vi "Measurement UI.vi"() -> ()   [LabVIEW 2021, in "ImageStreamRendering.lvlib"]
uses:
  ImageStreamRendering.lvlib
  <vilib>/vision/Image Controls.llb/IMAQ Image.ctl
  nivision.dll
  nivissvc.dll
panel:
  out "Image Res megapixel":dbl
  in  "External Display":bool
  out "Average Time to receive image frame":dbl
  out "Time taken to receive image frame":dbl
  out "Image Acq time":string
  out "Display Frames per Second (approx)":u32
  out "Last Buffer Number":u32
  out "Time to convert back to Image (s)":dbl
  in  "Border Size":i32=3
  in  "Image Name":string="copy"
  in  "Image Type":u32(ring)=4 items=["Grayscale (U8)", "Grayscale (I16)", "Grayscale (SGL)", "Complex (CSG)", "RGB (U32)", "HSL (U32)", "RGB (U64)", "Grayscale (U16)"]
  out "Image Resolution":i32[](array[numeric])
  in  "Camera name":string
  out "Image Pixels (U32)":u32[](array[numeric])
  in  "Image Pixels (U64) 2":T1[][](array[typedef])
  in  "Image Converison Type":string(combo)="ImagePixelArray"
  out "Image Data Received":string
  out "value":u32[][](array[numeric])
  out "Image":T2(plugin-control)
  out "error out":errorcluster
  out "Image Data":string
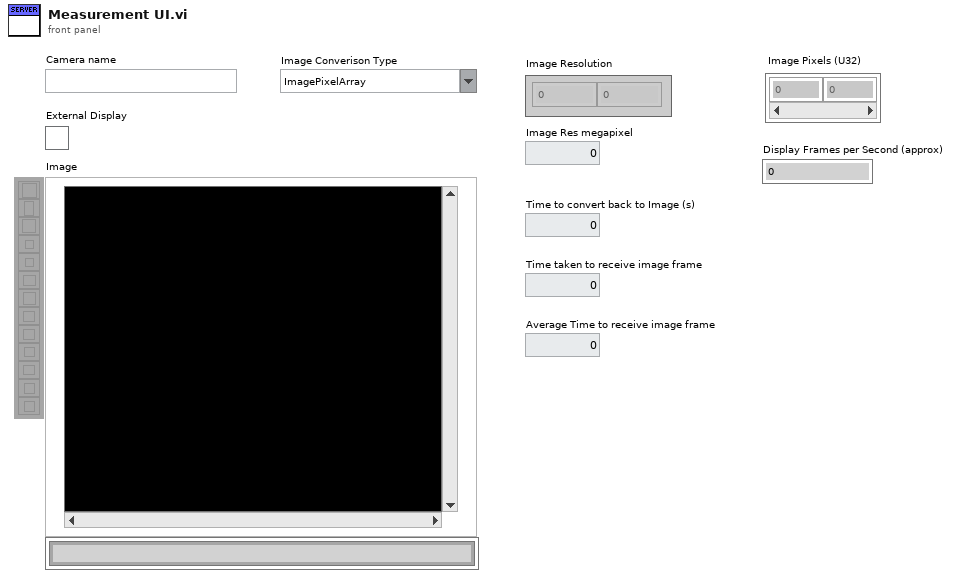
[diagram p1: front panel]
types:
  T1 = typedef "Color (U64)" = cluster{"Plane 3 (Blue)":u16, "Plane 2 (Green)":u16, "Plane 1 (Red)":u16, "Plane 4 (alpha)":u16}
  T2 = typedef "IMAQ Image.ctl" = refnum<image>
  T3 = cluster{"New Image":T2, "Run start time":timestamp, "Last Buffer Number":u32, "Time to receive image":dbl[]}
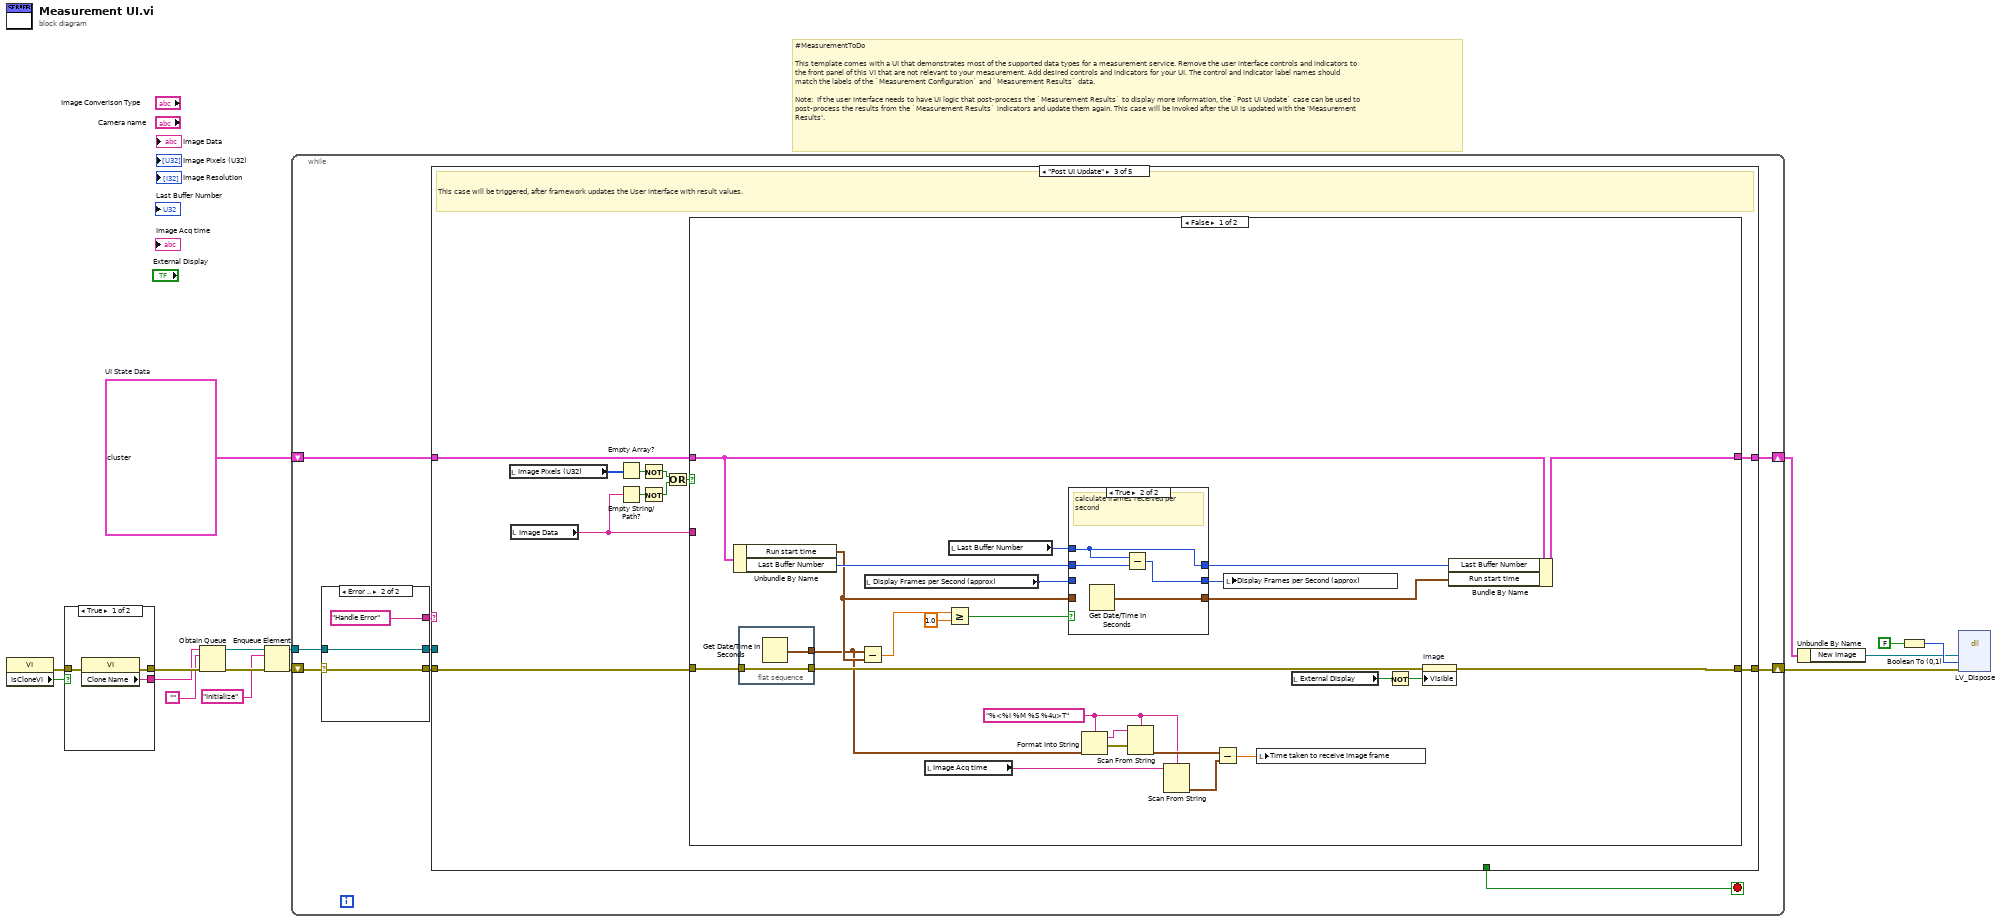
[diagram p0: block diagram]
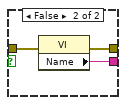
[diagram p2: hidden frame]
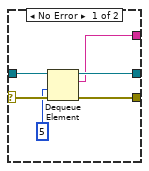
[diagram p3: hidden frame]
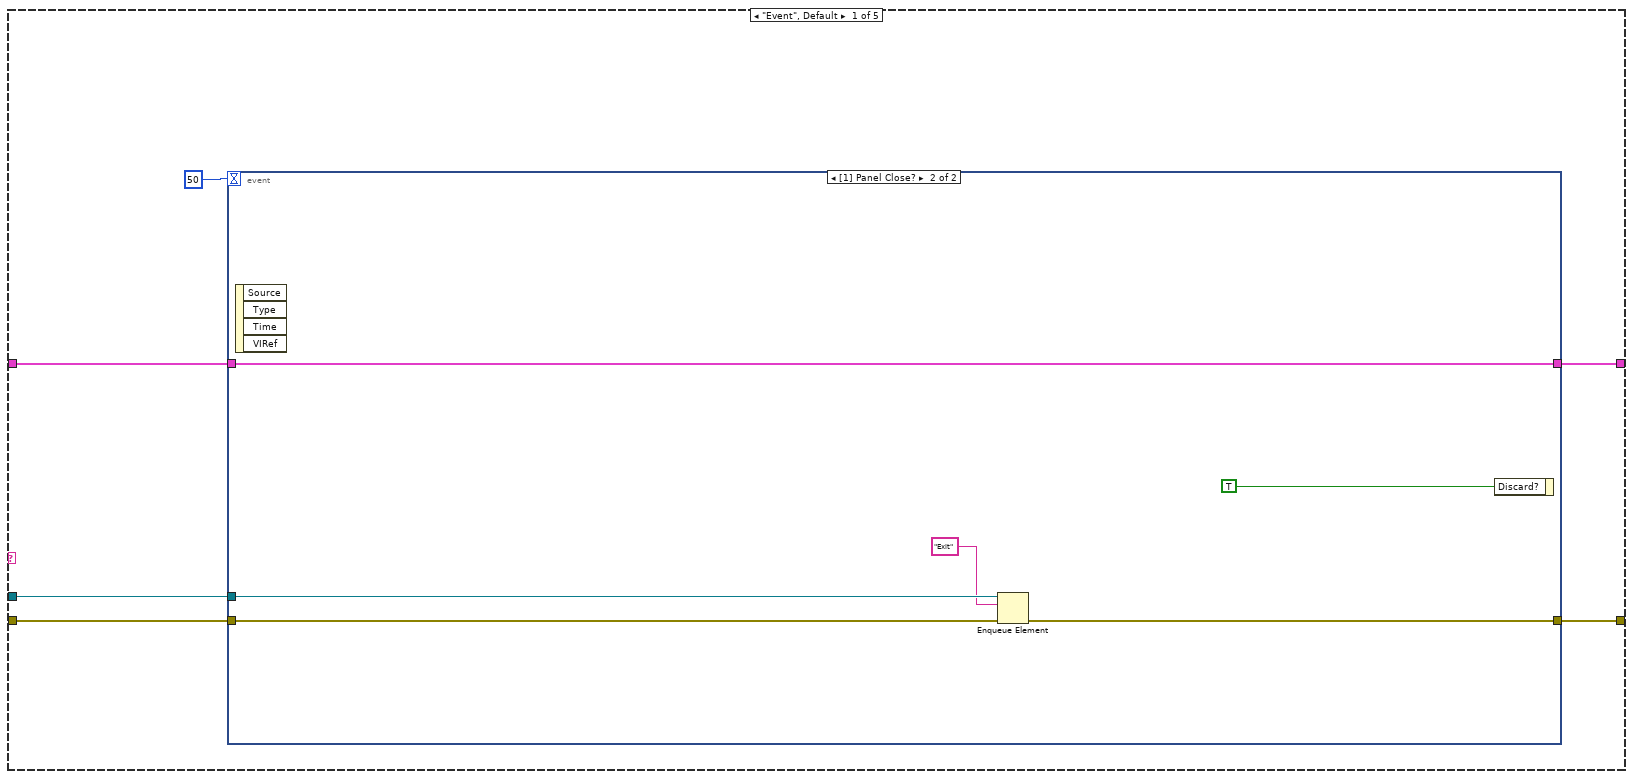
[diagram p4: hidden frame]
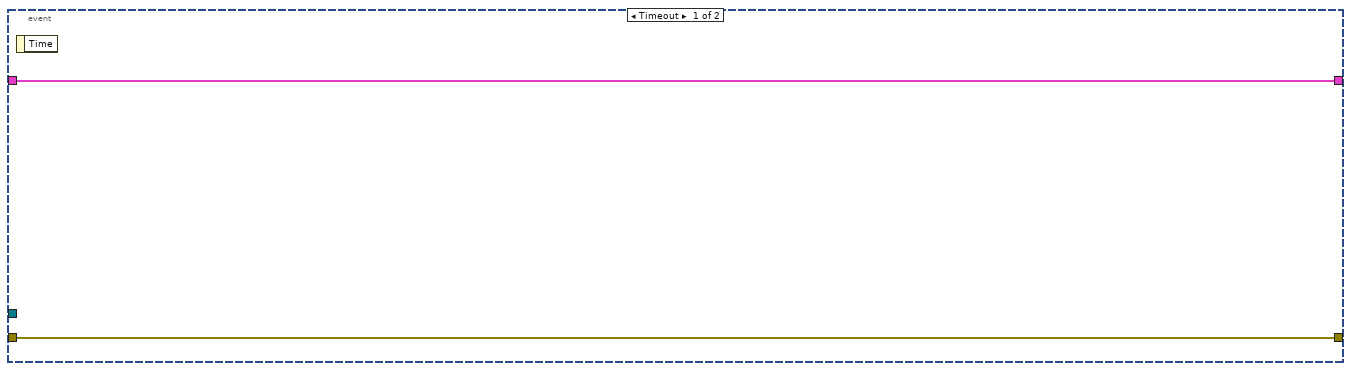
[diagram p5: hidden frame]
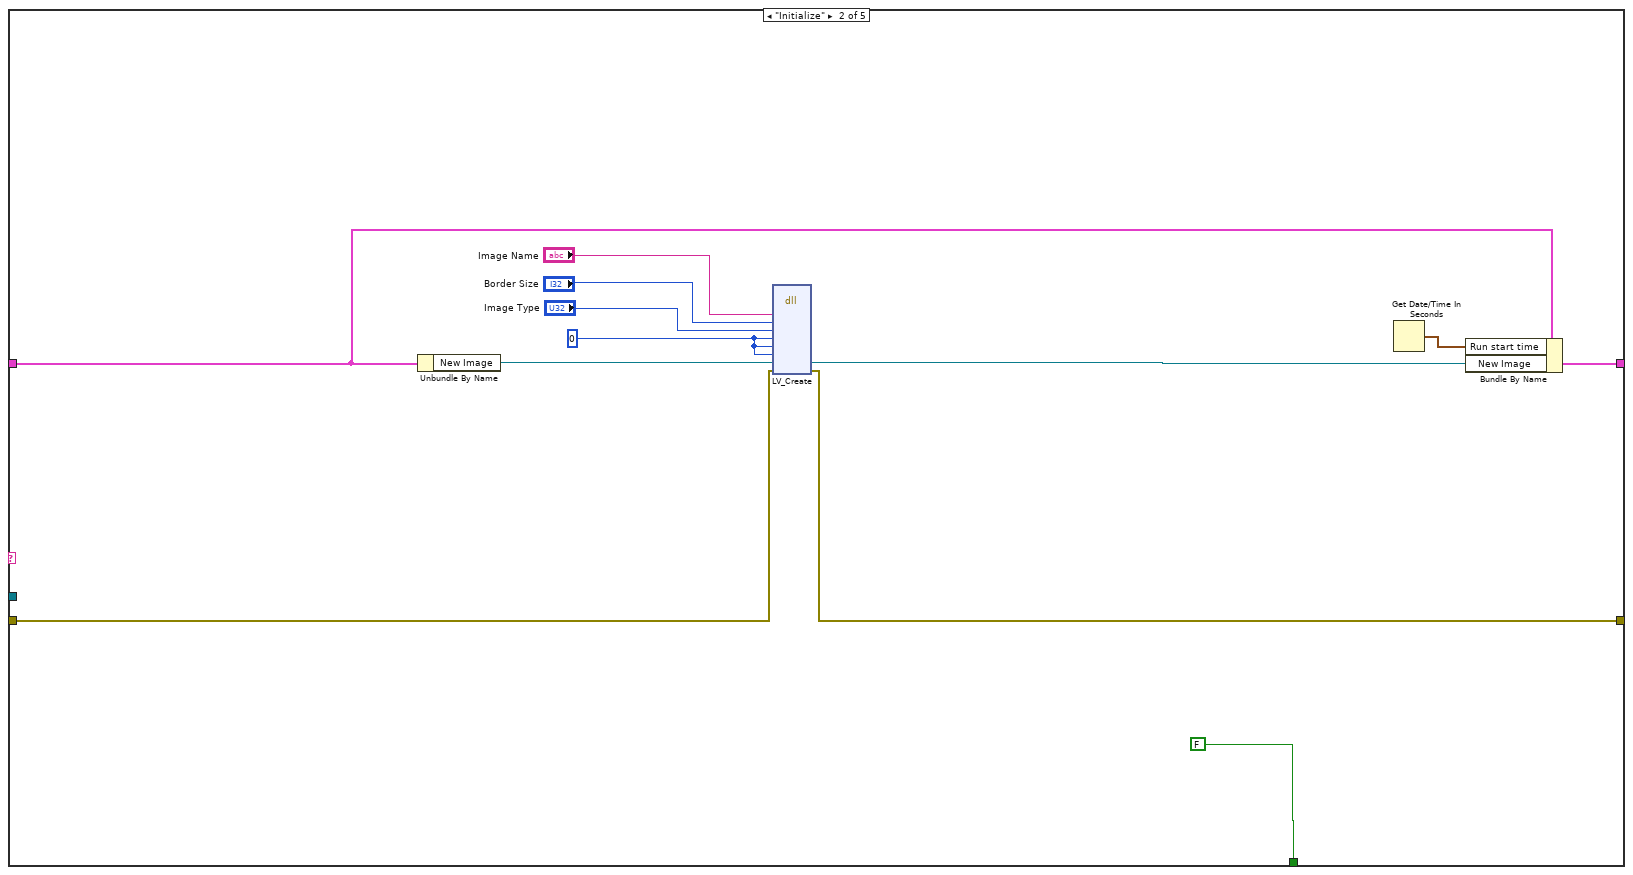
[diagram p6: hidden frame]
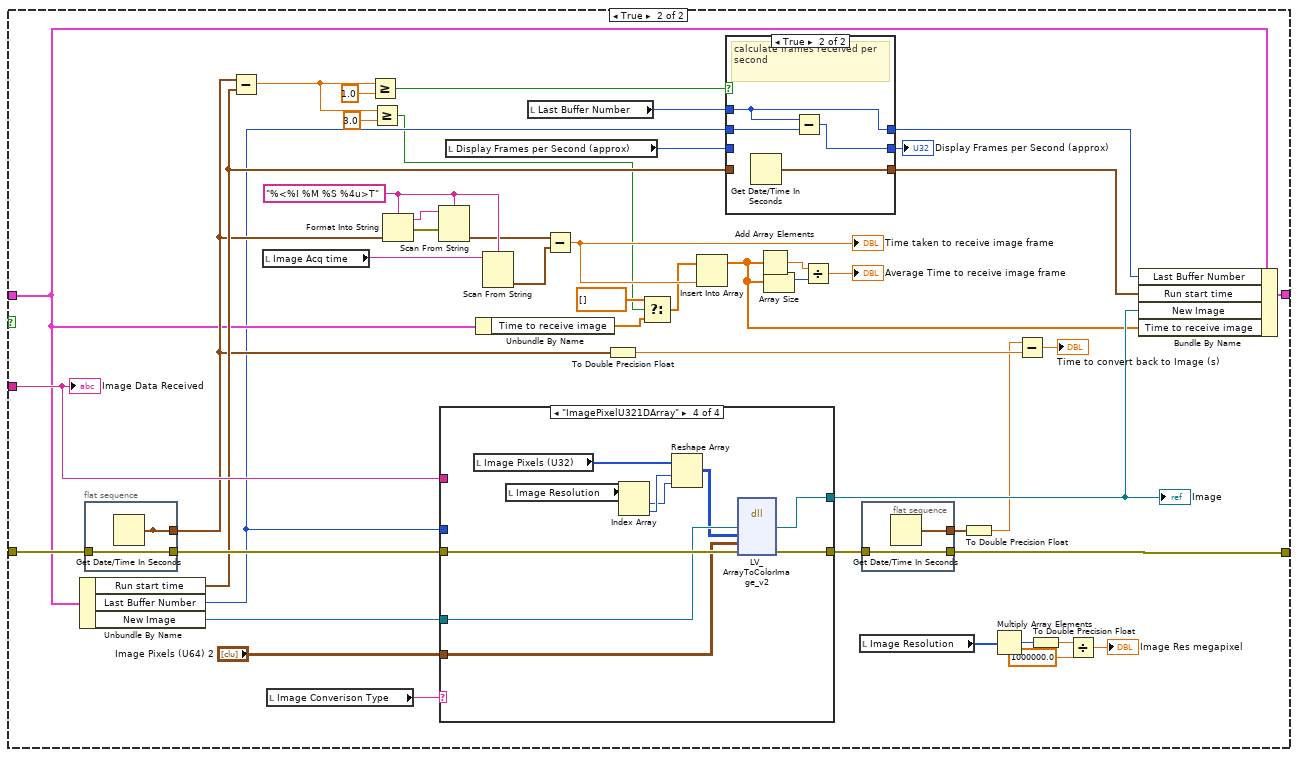
[diagram p8: hidden frame]
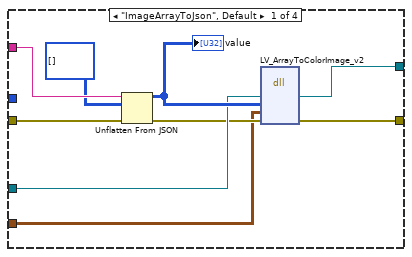
[diagram p10: hidden frame]
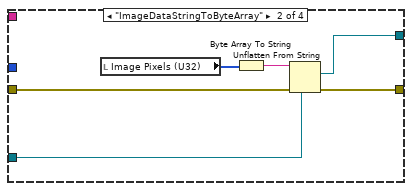
[diagram p11: hidden frame]
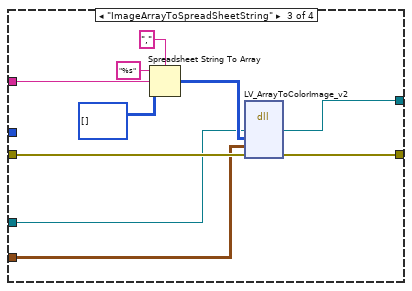
[diagram p12: hidden frame]
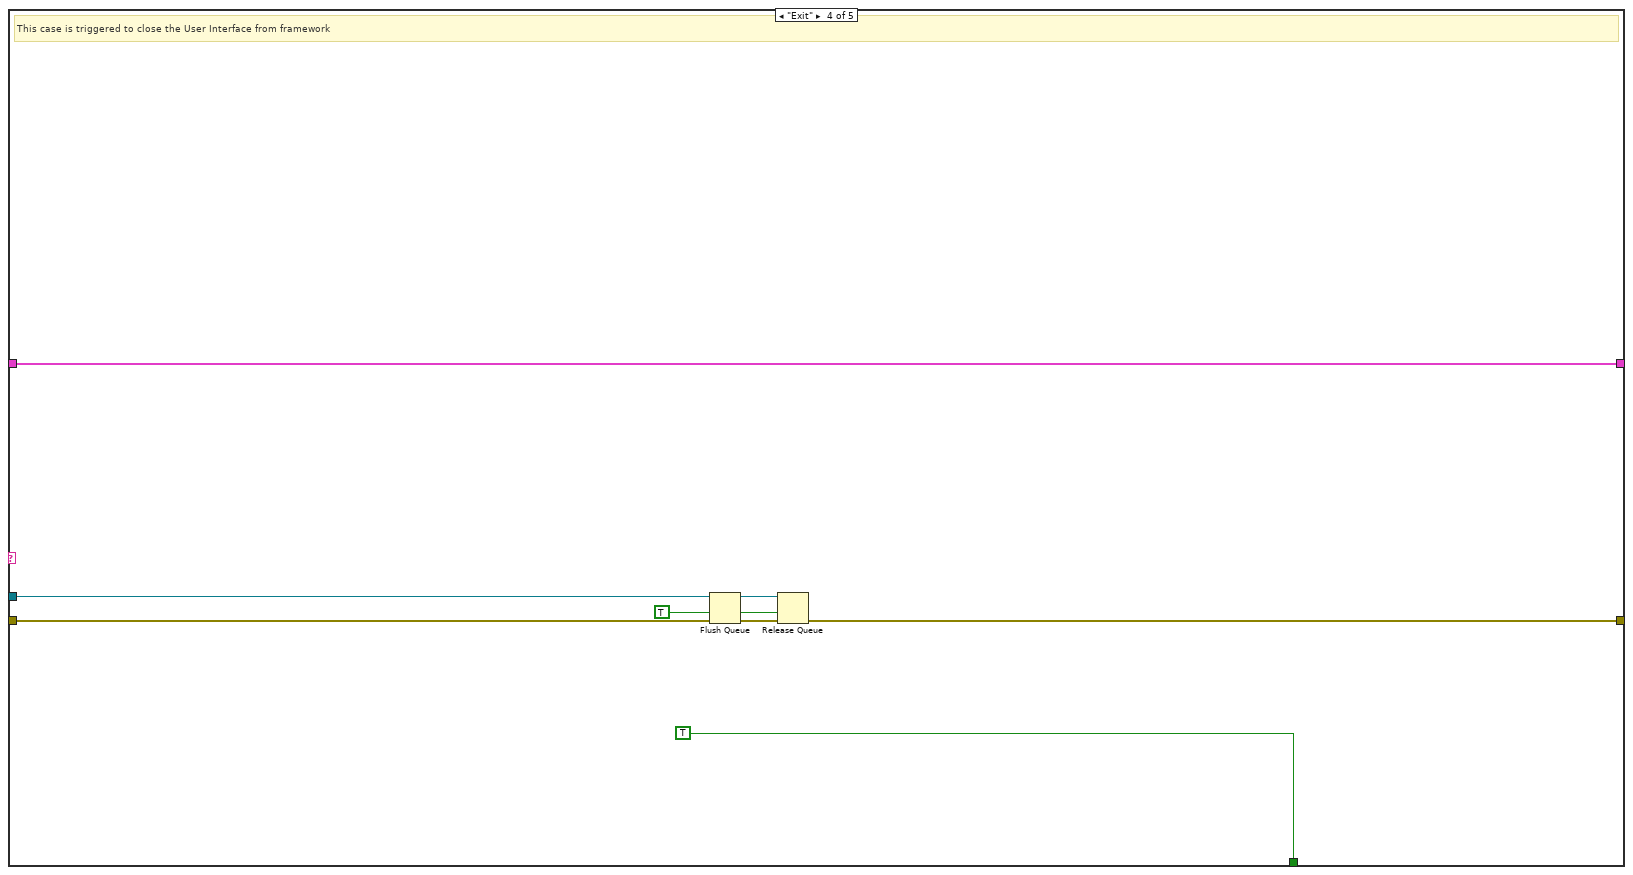
[diagram p13: hidden frame]
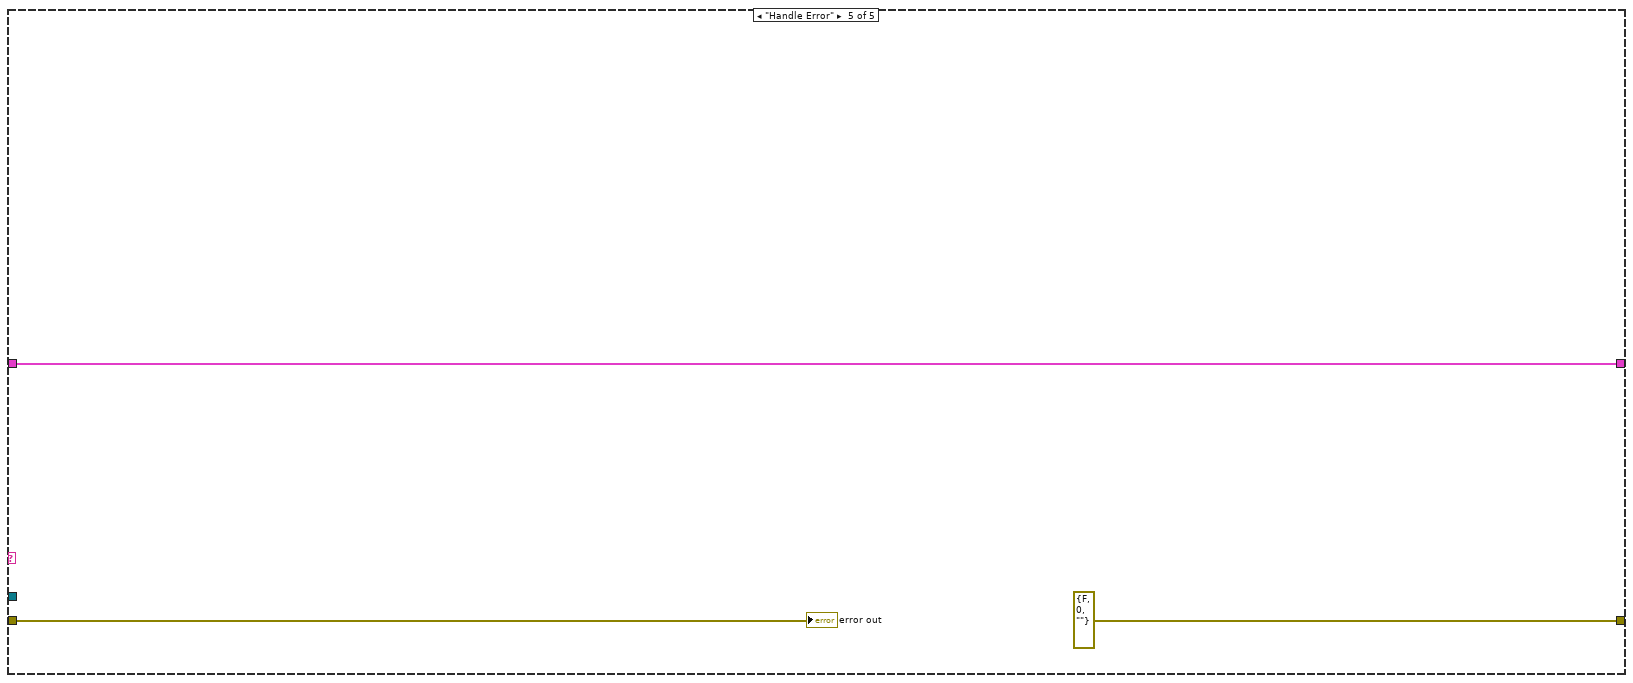
[diagram p14: hidden frame]
diagram:
  w2 = T3 {"New Image"=refnum, "Run start time"=timestamp(0 s since 1904-01-01), "Last Buffer Number"=0, "Time to receive image"=[]}  # UI State Data
  # "#MeasurementToDo  \n\nThis template comes with a UI that demonstrates most of the supported data types for a measurement service. Remove the user interface controls and indicators to the front panel of this VI that are not relevant to your measurement. Add desired controls and indicators for your UI. The control and indicator label names should match the labels of the `Measurement Configuration` and `Measurement Results` data.\n\nNote:  If the user interface needs to have UI logic that post-process the `Measurement Results` to display more information, the `Post UI Update` case can be used to post-process the results from the `Measurement Results` indicators and update them again. This case will be invoked after the UI is updated with the 'Measurement Results'."
  n1 = property class="VI"() -> (error out=w7:errorcluster, "IsCloneVI"=w8:bool)  [unwired: 2 in, 1 out]
  n2 = case shown="True" w8 {
    tunnel: [w19 w22] -> w16
    tunnel: [w18 w21] -> w15
    tunnel: w7 -> [w17 w20]
    frame True {
      n3 = property class="VI"(error in=w17) -> (error out=w19:errorcluster, "Clone Name"=w18:string)  [unwired: 1 in, 1 out]
    }
    frame False {
      n4 = property class="VI"(error in=w20) -> (error out=w22:errorcluster, "Name"=w21:string)  [unwired: 1 in, 1 out]
    }
  }
  n5 = Obtain Queue(name (unnamed)=w15, element data type="", error in (no error)=w16) -> (queue out=w12:refnum<queue>, error out=w14:errorcluster)  [unwired: 2 in, 1 out]
  n6 = Enqueue Element(queue=w12, element="Initialize", error in (no error)=w14) -> (queue out=w11:refnum<queue>, error out=w13:errorcluster)  [unwired: 1 in, 1 out]
  n7 = while {
    shift-right: [w27] -> w5
    shift-left: w13 -> [w31]
    tunnel: w11 -> [w30]
    shift-right: [w24] -> w3
    shift-left: w2 -> [w23]
    stop <- w26 stop-if-true
    n8 = case shown="Error .." w31 {
      selector: w31 -> [w37 w40]
      tunnel: [w36 w40] -> w25
      tunnel: w30 -> [w35 w39]
      tunnel: [w34 w39] -> w29
      tunnel: [w33 "Handle Error"] -> w28
      frame No Error {
        n9 = Dequeue Element(queue=w35, timeout in ms (-1)=5, error in (no error)=w37) -> (queue out=w34:refnum<queue>, element=w33:string, error out=w36:errorcluster)  [unwired: 1 out]
      }
      frame Error {
      }
    }
    n10 = case shown="\"Post UI Update\"" w28 {
      tunnel: w25 -> [w45 w61 w67 w212 w215]
      tunnel: w29 -> [w43 _ _ w210 _]
      tunnel: [w46 w55 w77 w207 errorcluster {"status"=FALSE, "code"=0, "source"=""} ("error out")] -> w27
      tunnel: [_ FALSE _ TRUE _] -> w26
      tunnel: [w41 w58 w69 w205 w214] -> w24
      tunnel: w23 -> [w42 w57 w68 w205 w214]
      frame "Event", Default {
        n11 = event shown="[1] Panel Close?" {
          selector: _ -> [_ _]
          dyn-events: _ -> [_ _]
          timeout: 50 -> [_ _]
          tunnel: [w48 w52] -> w46
          tunnel: w45 -> [w48 w53]
          tunnel: w43 -> [_ w51]
          tunnel: w42 -> [w47 w49]
          tunnel: [w47 w49] -> w41
          event Timeout {
            n12 = event-data() -> ()  [unwired: 1 in, 1 out]
          }
          event Panel Close? {
            n13 = event-data() -> ()  [unwired: 1 in, 4 out]
            n14 = Enqueue Element(queue=w51, element="Exit", error in (no error)=w53) -> (error out=w52:errorcluster)  [unwired: 1 in, 2 out]
            n15 = event-data("Discard?"=TRUE) -> ()  [unwired: 1 in, 1 out]
          }
        }
      }
      frame "Initialize" {
        w62 = 0
        n16 = Unbundle By Name(w57) -> ("New Image"=w59:T2)
        n17 = dll-call lib="nivissvc.*" fn="LV_Create" label="Imaq Create"("name"="Image Name", "border"="Border Size", "imageType"="Image Type", "width"=w62, "height"=w62, "lock space"=w62, "image"=w59, "error out 2"=w61) -> ("image"=w60:T2, "error out 2"=w55:errorcluster)  [unwired: 9 in, 3 out]
        n18 = Get Date/Time In Seconds() -> (seconds since 1Jan1904=w56:timestamp)
        n19 = Bundle By Name(cluster=w57, "Run start time"=w56, "New Image"=w60) -> (w58:T3)
      }
      frame "Post UI Update" {
        # "This case will be triggered, after framework updates the User interface with result values."
        n20 = local read "Image Pixels (U32)"() -> (w75:u32[])
        n21 = local read "Image Data"() -> (w73:string)
        n22 = Empty Array?(array=w75) -> (empty?=w76:bool)
        n23 = Empty String/Path?(string/path=w73) -> (empty?=w72:bool)
        n24 = Not(x=w76) -> (.not. x?=w74:bool)
        n25 = Not(x=w72) -> (.not. x?=w71:bool)
        n26 = Or(x=w74, y=w71) -> (x .or. y?=w70:bool)
        n27 = case shown="False" w70 {
          tunnel: [w100 w153] -> w77
          tunnel: w67 -> [w98 w157]
          tunnel: w73 -> [_ w155]
          tunnel: [w88 w149] -> w69
          tunnel: w68 -> [w99 w128]
          frame False {
            w81 = "%<%I %M %S %4u>T" ("format string")
            n28 = Unbundle By Name(w99) -> ("Run start time"=w92:timestamp, "Last Buffer Number"=w96:u32)
            n29 = flat-sequence {
              tunnel: w98 -> [w104]
              tunnel: [w104] -> w97
              tunnel: [w103] -> w79
              frame #0 {
                n30 = Get Date/Time In Seconds() -> (seconds since 1Jan1904=w103:timestamp)
              }
            }
            n31 = Subtract(x=w79, y=w92) -> (x-y=w94:dbl)
            n32 = local read "Display Frames per Second (approx)"() -> (w90:u32)
            n33 = local read "Image Acq time"() -> (w80:string)
            n34 = Greater Or Equal?(x=w94, y=1.0) -> (x >= y?=w93:bool)
            n35 = local read "Last Buffer Number"() -> (w91:u32)
            n36 = case shown="True" w93 {
              tunnel: w96 -> [w105 w111]
              tunnel: [w107 w110] -> w86
              tunnel: w92 -> [w107 _]
              tunnel: [w106 w109] -> w89
              tunnel: w90 -> [w106 _]
              tunnel: w91 -> [_ w108]
              tunnel: [w105 w108] -> w87
              frame False {
              }
              frame True {
                # "calculate frames received per second"
                n37 = Get Date/Time In Seconds() -> (seconds since 1Jan1904=w110:timestamp)
                n38 = Subtract(x=w108, y=w111) -> (x-y=w109:u32)
              }
            }
            n39 = Format Into String(format string=w81, w79) -> (resulting string=w83:string, error out=w84:errorcluster)  [unwired: 2 in]
            n40 = Scan From String(format string=w81, input string=w83, error in=w84) -> (output 1=w82:timestamp)  [unwired: 2 in, 3 out]
            n41 = Scan From String(format string=w81, input string=w80) -> (output 1=w85:timestamp)  [unwired: 3 in, 3 out]
            n42 = Subtract(x=w82, y=w85) -> (x-y=w78:dbl)
            n43 = local write "Display Frames per Second (approx)"(w89) -> ()
            n44 = local write "Time taken to receive image frame"(w78) -> ()
            n45 = local read "External Display"() -> (w101:bool)
            n46 = Not(x=w101) -> (.not. x?=w102:bool)
            n47 = property on="Image" class="ImageControl"(error in=w97, "Visible"=w102) -> (error out=w100:errorcluster)  [unwired: 1 in, 1 out]
            n48 = Bundle By Name(cluster=w99, "Last Buffer Number"=w87, "Run start time"=w86) -> (w88:T3)
          }
          frame True {
            w138 = "%<%I %M %S %4u>T" ("format string")
            n49 = Unbundle By Name(w128) -> ("Run start time"=w144:timestamp, "Last Buffer Number"=w125:u32, "New Image"=w132:T2)
            n50 = flat-sequence {
              tunnel: w157 -> [w202]
              tunnel: [w202] -> w152
              tunnel: [w201] -> _
              tunnel: [w201] -> w133
              frame #0 {
                n51 = Get Date/Time In Seconds() -> (seconds since 1Jan1904=w201:timestamp)
              }
            }
            n52 = Subtract(x=w133, y=w144) -> (x-y=w117:dbl)
            n53 = local read "Image Acq time"() -> (w142:string)
            n54 = local read "Image Converison Type"() -> (w156:string)
            n55 = Greater Or Equal?(x=w117, y=1.0) -> (x >= y?=w147:bool)
            n56 = Greater Or Equal?(x=w117, y=3.0) -> (x >= y?=w113:bool)
            n57 = Format Into String(format string=w138, w133) -> (resulting string=w139:string, error out=w140:errorcluster)  [unwired: 2 in]
            n58 = Scan From String(format string=w138, input string=w139, error in=w140) -> (output 1=w137:timestamp)  [unwired: 2 in, 3 out]
            n59 = case shown="\"ImagePixelU321DArray\"" w156 {
              tunnel: w155 -> [w174 _ w190 _]
              tunnel: w132 -> [w171 w178 w183 w198]
              tunnel: [w170 w177 w182 w197] -> w131
              tunnel: [w169 w179 w186 w199] -> w158
              tunnel: w152 -> [w168 w180 w187 w200]
              tunnel: "Image Pixels (U64) 2" -> [w166 _ w181 w196]
              tunnel: w125 -> [_ _ _ _]
              frame "ImageArrayToJson", Default {
                n60 = Unflatten From JSON(JSON string=w174, type and defaults=u32[][] [] ("Image Pixels (U32)"), error in (no error)=w168) -> (value=w172:u32[][], error out=w167:errorcluster)  [unwired: 4 in]
                "value" <- w172
                n61 = dll-call lib="nivision.*" fn="LV_ArrayToColorImage_v2"("image"=w171, "array32"=w172, "array64"=w166, "error"=w167) -> ("image"=w170:T2, "error"=w169:errorcluster)  [unwired: 5 in, 3 out]
              }
              frame "ImageDataStringToByteArray" {
                n62 = local read "Image Pixels (U32)"() -> (w176:u32[])
                n63 = Byte Array To String(unsigned byte array=w176) -> (string=w175:string)
                n64 = Unflatten From String(type=w178, binary string=w175, error in (no error)=w180) -> (value=w177:T2, error out=w179:errorcluster)  [unwired: 2 in, 1 out]
              }
              frame "ImageArrayToSpreadSheetString" {
                n65 = Spreadsheet String To Array(delimiter (Tab)=",", format string="%s", spreadsheet string=w190, array type (2D Dbl)=u32[][] [] ("Image Pixels (U32)")) -> (array=w185:u32[][])
                n66 = dll-call lib="nivision.*" fn="LV_ArrayToColorImage_v2"("image"=w183, "array32"=w185, "array64"=w181, "error"=w187) -> ("image"=w182:T2, "error"=w186:errorcluster)  [unwired: 5 in, 3 out]
              }
              frame "ImagePixelU321DArray" {
                n67 = local read "Image Pixels (U32)"() -> (w195:u32[])
                n68 = local read "Image Resolution"() -> (w194:i32[])
                n69 = Index Array(array=w194) -> (element #1=w192:i32, element #2=w193:i32)  [unwired: 2 in]
                n70 = Reshape Array(w195, w193, w192) -> (w191:u32[][])
                n71 = dll-call lib="nivision.*" fn="LV_ArrayToColorImage_v2"("image"=w198, "array32"=w191, "array64"=w196, "error"=w200) -> ("image"=w197:T2, "error"=w199:errorcluster)  [unwired: 5 in, 3 out]
              }
            }
            "Image" <- w131
            n72 = local read "Display Frames per Second (approx)"() -> (w145:u32)
            n73 = Unbundle By Name(w128) -> ("Time to receive image"=w115:dbl[])
            n74 = Scan From String(format string=w138, input string=w142) -> (output 1=w141:timestamp)  [unwired: 3 in, 3 out]
            n75 = local read "Last Buffer Number"() -> (w146:u32)
            n76 = Subtract(x=w137, y=w141) -> (x-y=w127:dbl)
            "Time taken to receive image frame" <- w127
            n77 = To Double Precision Float(number=w133) -> (double precision float=w119:dbl)
            n78 = Select(t=dbl[] [], s=w113, f=w115) -> (s? t:f=w112:dbl[])
            n79 = Insert Into Array(array=w112, new element=w127) -> (w126:dbl[])  [unwired: 1 in]
            n80 = case shown="True" w147 {
              tunnel: w125 -> [w159 w165]
              tunnel: [w161 w164] -> w129
              tunnel: w144 -> [w161 _]
              tunnel: [w160 w163] -> w143
              tunnel: w145 -> [w160 _]
              tunnel: w146 -> [_ w162]
              tunnel: [w159 w162] -> w130
              frame False {
              }
              frame True {
                # "calculate frames received per second"
                n81 = Get Date/Time In Seconds() -> (seconds since 1Jan1904=w164:timestamp)
                n82 = Subtract(x=w162, y=w165) -> (x-y=w163:u32)
              }
            }
            "Display Frames per Second (approx)" <- w143
            n83 = Add Array Elements(numeric array=w126) -> (sum=w136:dbl)
            n84 = Array Size(array=w126) -> (size(s)=w135:i32)
            n85 = Divide(x=w136, y=w135) -> (x/y=→"Average Time to receive image frame":dbl)
            n86 = local read "Image Resolution"() -> (w124:i32[])
            n87 = flat-sequence {
              tunnel: w158 -> [w204]
              tunnel: [w204] -> w153
              tunnel: [w203] -> w151
              frame #0 {
                n88 = Get Date/Time In Seconds() -> (seconds since 1Jan1904=w203:timestamp)
              }
            }
            n89 = To Double Precision Float(number=w151) -> (double precision float=w118:dbl)
            n90 = Multiply Array Elements(1:w124) -> (0:w123:i32)
            n91 = Subtract(x=w118, y=w119) -> (x-y=→"Time to convert back to Image (s)":dbl)
            n92 = To Double Precision Float(number=w123) -> (double precision float=w122:dbl)
            n93 = Divide(x=w122, y=1000000.0) -> (x/y=→"Image Res megapixel":dbl)
            n94 = Bundle By Name(cluster=w128, "Last Buffer Number"=w130, "Run start time"=w129, "New Image"=w131, "Time to receive image"=w126) -> (w149:T3)
            "Image Data Received" <- w155
          }
        }
      }
      frame "Exit" {
        # "This case is triggered to close the User Interface from framework"
        n95 = Flush Queue(queue=w210, error in (no error)=w212) -> (queue out=w209:refnum<queue>, error out=w208:errorcluster)  [unwired: 1 out]
        n96 = Release Queue(queue=w209, force destroy? (F)=TRUE, error in (no error)=w208) -> (error out=w207:errorcluster)  [unwired: 2 out]
      }
      frame "Handle Error" {
        "error out" <- w215
      }
    }
  }
  n97 = Unbundle By Name(w3) -> ("New Image"=w1:T2)
  n98 = Boolean To (0,1)(Boolean=FALSE) -> (0, 1=w6:i16)
  n99 = dll-call lib="nivissvc.*" fn="LV_Dispose"("image"=w1, "disposeAll"=w6, "err"=w5) -> ()  [unwired: 5 in, 4 out]
